vi "Autosort Delete pressed.vi"(9 "Data OUT":T1 {"Parameter Time Series"."time offset" format="%.3f"; "Parameter Time Series"."Gain" format="%.1f"; "Parameter Time Series"."Offset" format="%.1f"; "Parameter Time Series"."List 1" items=["Motor-Pos", "Motor-Vel", "Lx Position-in-Head", "Ly Position-in-Head", "Lz Position-in-Head", "Lx Velocity-in-Head", "Ly Velocity-in-Head", "Lz Velocity-in-Head", "Ll Velocity-in-Head", "Lr Velocity-in-Head", "Lx Accel-in-Head", "Ly Accel-in-Head", "Lz Accel-in-Head", "Rx Position-in-Head", "Ry Position-in-Head", "Rz Position-in-Head", "Rx Velocity-in-Head", "Ry Velocity-in-Head", "Rz Velocity-in-Head", "Rl Velocity-in-Head", "Rr Velocity-in-Head", "Rx Accel-in-Head", "Ry Accel-in-Head", "Rz Accel-in-Head", "Global Trigger", "", "", ""]; "Parameter Impuls Series"."Gain" format="%.1f"; "Parameter Impuls Series"."Offset" format="%.1f"}, 10 "reference":refnum<vi>, 11 "Ring in":refnum<vi>) -> ()   [LabVIEW 2013]
uses:
  type-defs/TD_Statemachine-Data.ctl
  type-defs/TD_Time Series.ctl
  type-defs/TD_Impulse Parameter.ctl
  plugins/Mars 3D/Mars3D_autosort.vi
  core.lvlib
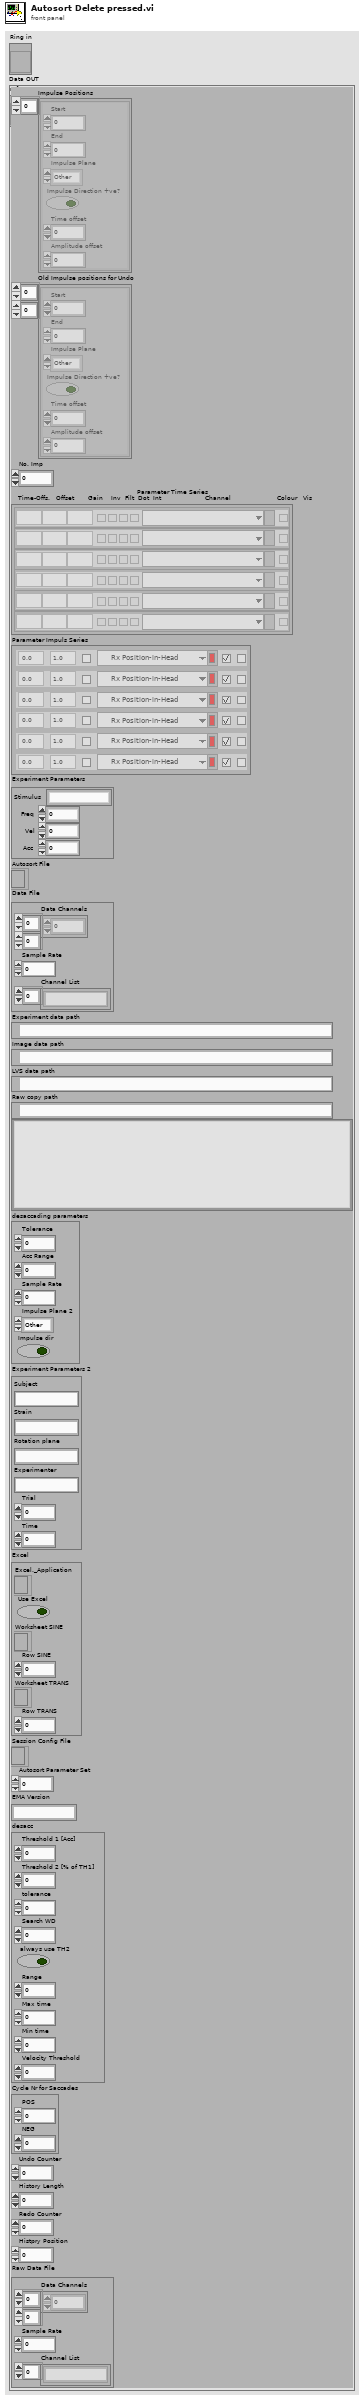
[diagram p1: front panel]
types:
  T1 = typedef "core.lvlib/TD_Statemachine-Data.ctl" = cluster{"Impulse Positions":cluster{"Start":i32, "End":i32, "Impulse Plane":enum16{"Other", "Yaw", "Pitch", "Roll", "LARP", "RALP"}, "Impulse Direction +ve?":bool, "Time offset":i32, "Amplitude offset":dbl}[], "Old Impulse positions for Undo":cluster{"Start":i32, "End":i32, "Impulse Plane":enum16{"Other", "Yaw", "Pitch", "Roll", "LARP", "RALP"}, "Impulse Direction +ve?":bool, "Time offset":i32, "Amplitude offset":dbl}[][], "No. Imp":i32, "Parameter Time Series":T2, "Parameter Impuls Series":T3, "Experiment Parameters":cluster{"Freq":dbl, "Vel":i32, "Acc":i32, "Stimulus":string}, "Autosort File":refnum<file>, "Data File":cluster{"Data Channels":dbl[][], "Sample Rate":i32, "Channel List":string[]}, "Experiment data path":path, "Image data path":path, "LVS data path":path, "Raw copy path":path, "filename":string, "desaccading parameters":cluster{"Tolerance":i32, "Acc Range":dbl, "Sample Rate":i32, "Impulse Plane 2":enum16{"Other", "Yaw", "Pitch", "Roll", "LARP", "RALP"}, "Impulse dir":bool}, "Experiment Parameters 2":cluster{"Subject":string, "Strain":string, "Rotation plane":string, "Experimenter":string, "Trial":dbl, "Time":dbl}, "Excel":cluster{"Excel._Application":refnum<k7>, "Use Excel":bool, "Worksheet SINE":refnum<k7>, "Row SINE":i32, "Worksheet TRANS":refnum<k7>, "Row TRANS":i32}, "Session Config File":refnum<file>, "Autosort Parameter Set":i32, "EMA Version":string, "desacc ":cluster{"Threshold 1 [Acc]":dbl, "Threshold 2 [% of TH1]":i32, "tolerance":i32, "Search WD ":dbl, " always use TH2":bool, "Range":dbl, "Max time":dbl, "Min time":dbl, "Velocity Threshold":i32}, "Cycle Nr for Saccades":cluster{"POS":i32, "NEG":i32}, "Undo Counter":i32, "History Length":i32, "Redo Counter":i32, "Histpry Position":i32, "Raw Data File":cluster{"Data Channels":dbl[][], "Sample Rate":i32, "Channel List":string[]}}
  T2 = typedef "core.lvlib/TD_Time Series.ctl" = cluster{"time offset":dbl, "Offset":dbl, "Gain":dbl, "inverse":bool, "filter data":bool, "dots":bool, "interpolate":bool, "List 1":u16, "Color Box":u32, "Boolean":bool}[]
  T3 = typedef "core.lvlib/TD_Impulse Parameter.ctl" = cluster{"Color":u32, "Visible":bool, "Channel":u16, "Invert":bool, "Desaccade":bool, "Offset":dbl, "Gain":dbl}[]
  T4 = cluster{"Autosize Parameter Set 2":cluster{"Trigger Ch":i32, "Min Vel":dbl, "MaxVel":dbl, "Width":i32, "Pre Impuls":i32, "Post Impuls":i32, "Pitch":dbl, "Name":string, "Other Trigger":bool, "Cross Corr":bool, "Default":cluster{"Freq":dbl, "Vel":dbl, "Acc":dbl, "Stimulus":string}}[]}[]
  T5 = cluster{"Autosize Parameter Set 2":cluster{"Trigger Ch":i32, "Min Vel":dbl, "MaxVel":dbl, "Width":i32, "Pre Impuls":i32, "Post Impuls":i32, "Pitch":dbl, "Name":string, "Other Trigger":bool, "Cross Corr":bool, "Default":cluster{"Freq":dbl, "Vel":dbl, "Acc":dbl, "Stimulus":string}}[]}
  T6 = cluster{"Trigger Ch":i32, "Min Vel":dbl, "MaxVel":dbl, "Width":i32, "Pre Impuls":i32, "Post Impuls":i32, "Pitch":dbl, "Name":string, "Other Trigger":bool, "Cross Corr":bool, "Default":cluster{"Freq":dbl, "Vel":dbl, "Acc":dbl, "Stimulus":string}}[]
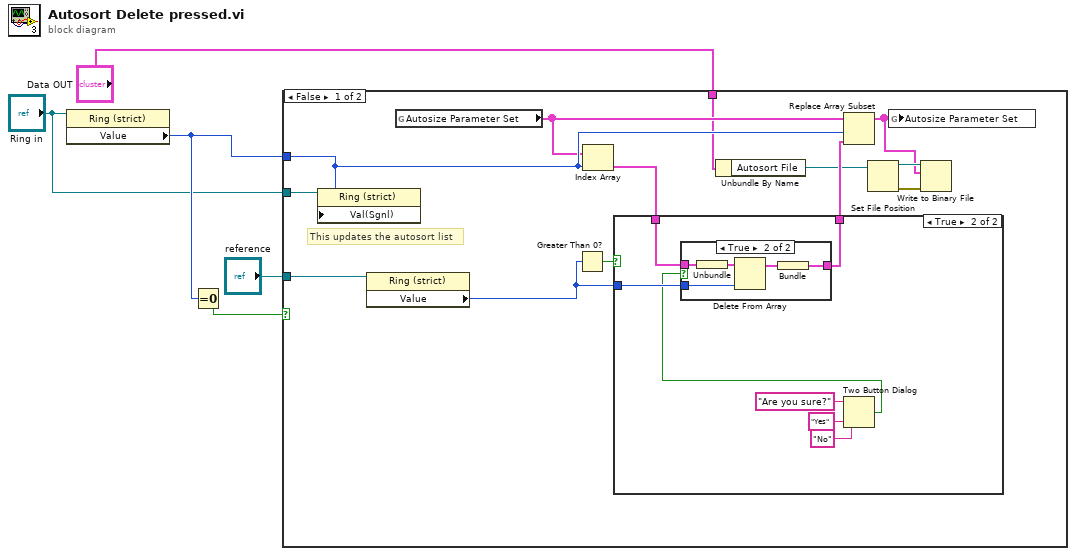
[diagram p0: block diagram]
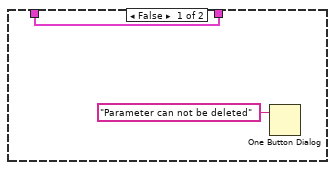
[diagram p2: hidden frame]
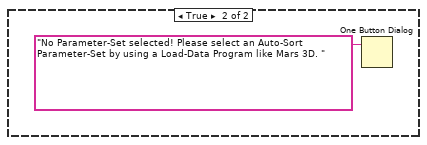
[diagram p4: hidden frame]
diagram:
  n1 = property on="Property Node" class="Ring (strict)"(reference="Ring in") -> ("Value"=w4:i8)  [unwired: 1 in, 2 out]
  n2 = Equal To 0?(x=w4) -> (x = 0?=w3:bool)
  n3 = case shown="False" w3 {
    tunnel: w4 -> [w18 _]
    tunnel: "Data OUT" -> [w9 _]
    tunnel: "Ring in" -> [w7 _]
    tunnel: "reference" -> [w6 _]
    frame False {
      # "This updates the autosort list"
      n4 = property on="Property Node" class="Ring (strict)"(reference=w7, "Val(Sgnl)"=w18) -> ()  [unwired: 1 in, 2 out]
      n5 = property class="Ring (strict)"(reference=w6) -> ("Value"=w13:u16)  [unwired: 1 in, 2 out]
      n6 = global read "Mars3D_autosort.vi" "Autosize Parameter Set"() -> (w17:T4)
      n7 = Greater Than 0?(x=w13) -> (x > 0?=w14:bool)
      n8 = Index Array(array=w17, index=w18) -> (element=w16:T5)
      n9 = case shown="True" w14 {
        tunnel: w16 -> [w20 w27]
        tunnel: [w20 w26] -> w15
        tunnel: w13 -> [_ w25]
        frame False {
          n10 = One Button Dialog(message="Parameter can not be deleted") -> ()  [unwired: 1 in, 1 out]
        }
        frame True {
          n11 = Two Button Dialog(message="Are you sure?", 1:"No" ("F button name (\"Cancel\")"), 2:"Yes" ("T button name (\"OK\")")) -> (T button?=w21:bool)
          n12 = case shown="True" w21 {
            tunnel: w27 -> [w28 w33]
            tunnel: [w28 w32] -> w26
            tunnel: w25 -> [_ w30]
            frame False {
            }
            frame True {
              n13 = Unbundle(w33) -> ("Autosize Parameter Set 2"=w31:T6)
              n14 = Delete From Array(array=w31, index=w30) -> (array with subset deleted=w29:T6)  [unwired: 1 in, 1 out]
              n15 = Bundle("Autosize Parameter Set 2"=w29) -> (w32:T5)  [unwired: 1 in]
            }
          }
        }
      }
      n16 = Unbundle By Name(w9) -> ("Autosort File"=w8:refnum<file>)
      n17 = Replace Array Subset(array=w17, new element=w15, index=w18) -> (w10:T4)
      n18 = Set File Position(refnum=w8) -> (refnum out=w11:refnum<file>, error out=w12:errorcluster)  [unwired: 3 in]
      n19 = global write "Mars3D_autosort.vi" "Autosize Parameter Set"(w10) -> ()
      n20 = Write to Binary File(file (use dialog)=w11, data=w10, error in=w12) -> ()  [unwired: 3 in, 3 out]
    }
    frame True {
      n21 = One Button Dialog(message="No Parameter-Set selected! Please select an Auto-Sort Parameter-Set by using a Load-Data Program like Mars 3D. ") -> ()  [unwired: 1 in, 1 out]
    }
  }
